vi "Find Scalar in Section.vi"(8 "error in":errorcluster, 10 "Scalar Data":T5, 11 "FPGA Addon refnum in":T2 format="%.0x") -> (0 "error out":errorcluster, 1 "Found ?":bool, 2 "Section Scalar Data":T1 {"Register Information"."Data Type" format="%.0x"; "Scalar Section ref" format="%.0x"}, 3 "FPGA Addon refnum out":T2=18446744073709551615 format="%.0x")   [LabVIEW 2018, in "Scripting API.lvlib"]
uses:
  Scripting API.lvlib
  <vilib>/NI Veristand/Custom Device API/Custom Device Item Ref.ctl
  TypeDefs/Input Scalar Data.ctl
  TypeDefs/Section Scalar Data.ctl
  Addon/Addon Shared/Types/Register Information.ctl
  Addon/Addon Shared/Types/FPGA Addon Data Type.ctl
  Addon/Addon Shared/Types/FG Action.ctl
  Addon/Addon Shared/SubVIs/Constants.vi
  <vilib>/NI/NI VeriStand Advanced SysDef API/_SubVIs/SysDef.Search.GUID.vi
  <vilib>/NI/NI VeriStand Advanced SysDef API/SysDef API/SysDef.Property.Get.vi
  <vilib>/NI/NI VeriStand Advanced SysDef API/_SubVIs/SysDef.Property.Get.Variant.vi
  <vilib>/NI/NI VeriStand Advanced SysDef API/SysDef API/SysDef.Property.Set.vi
  <vilib>/NI/NI VeriStand Advanced SysDef API/_SubVIs/SysDef.Property.Set.Variant.vi
  <vilib>/NI/NI VeriStand Advanced SysDef API/SysDef API/Advanced System Definition.lvlib
  Addon/Addon Shared/FPGA Addon Shared.lvlib
  <vilib>/NI Veristand/Custom Device API/Custom Device API.lvlib
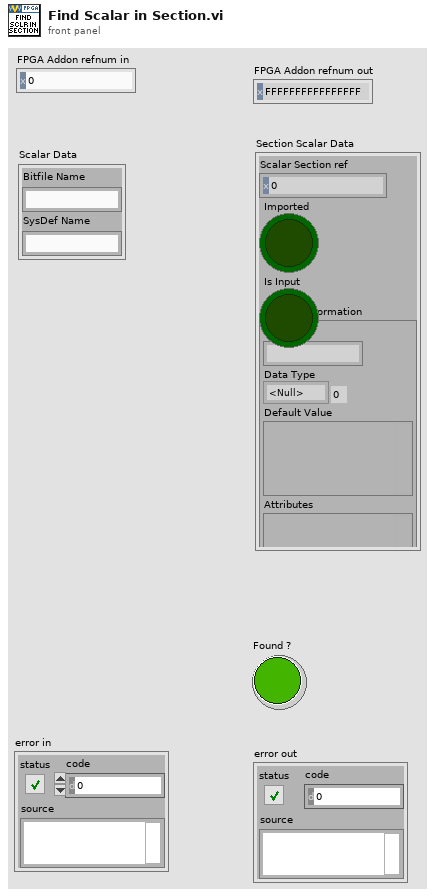
[diagram p1: front panel]
types:
  T1 = typedef "Scripting API.lvlib/Section Scalar Data.ctl" = cluster{"Scalar Section ref":T2, "Imported":bool, "Is Input":bool, "Register Information":T3}
  T2 = typedef "Custom Device API.lvlib/Custom Device Item Ref.ctl" = u64
  T3 = typedef "FPGA Addon Shared.lvlib/Register Information.ctl" = cluster{"Name":string, "Data Type":T4, "Default Value":variant, "Attributes":variant}
  T4 = typedef "FPGA Addon Shared.lvlib/FPGA Addon Data Type.ctl" = enum8{"<Null>", "I8", "I16", "I32", "I64", "U8", "U16", "U32", "U64", "SGL", "Boolean", "Analog PWM In Settings", "Analog PWM In", "Digital PWM In Settings", "Digital PWM In", "Digital PWM Out", "Sine Out", "FXP", "FXP+/-24.5", "FXP+/-16.5", "FXP+/-32.8", "FXP+/-64.32", "FXP+/-16.7", "FXP+/-20.5", "FXP+/-27.5", "FXP+/-32.16", "FXP+16.3", "FXP+18.3", "Digital Static In", "Digital Static Out", "Digital Static In Settings", "Digital WSS Out", "Quad Encoder Settings", "Quad Encoder In", "Group"}
  T5 = typedef "Scripting API.lvlib/Input Scalar Data.ctl" = cluster{"Bitfile Name":string, "SysDef Name":string}
  T6 = typedef "FPGA Addon Shared.lvlib/FG Action.ctl" = enum8{"GET", "SET"}
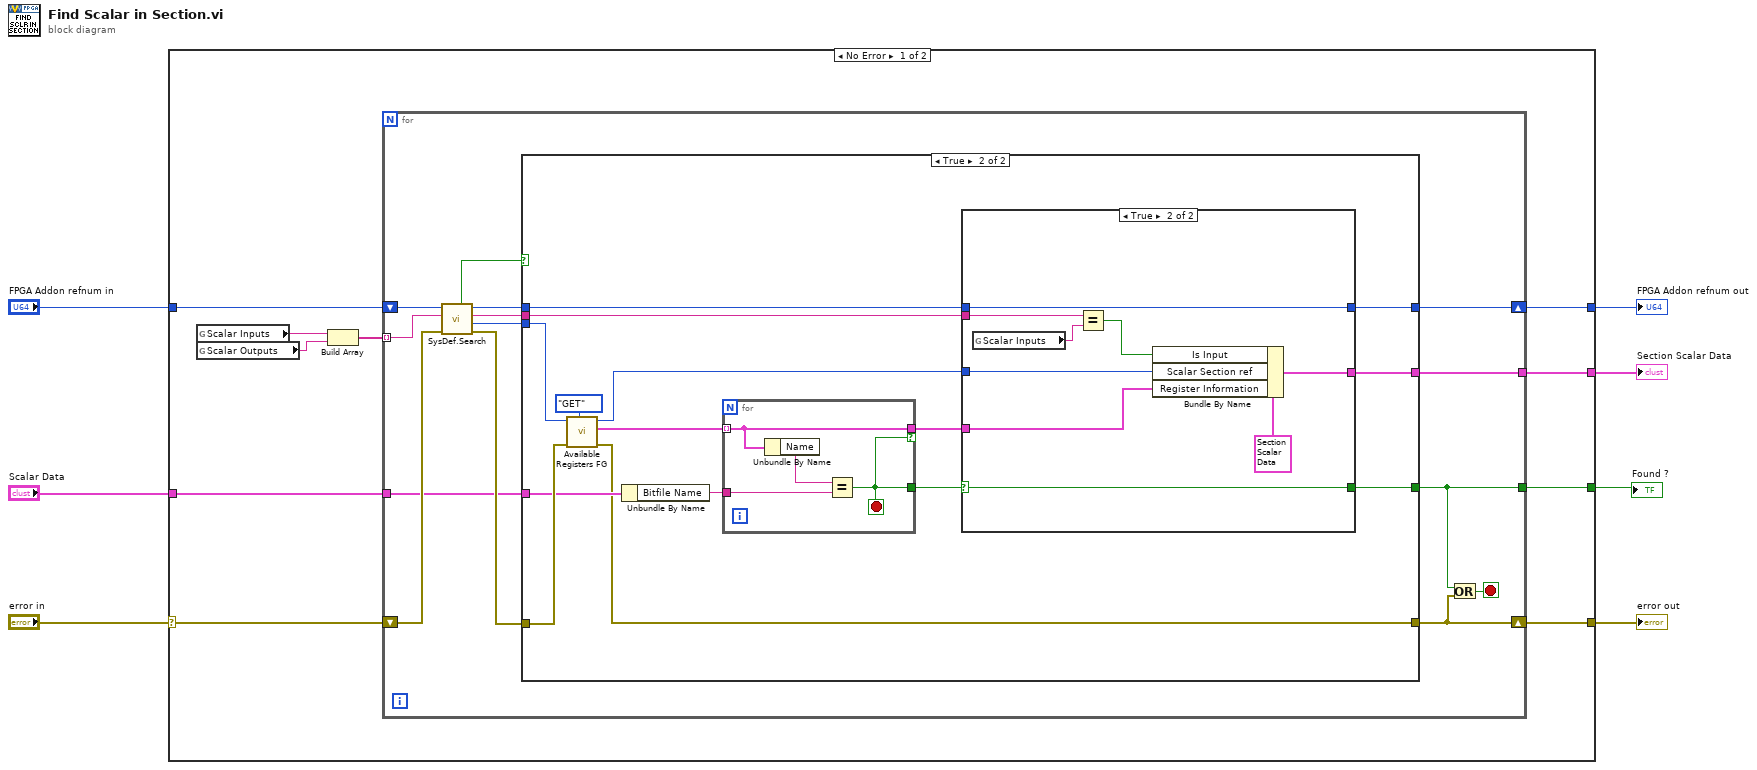
[diagram p0: block diagram]
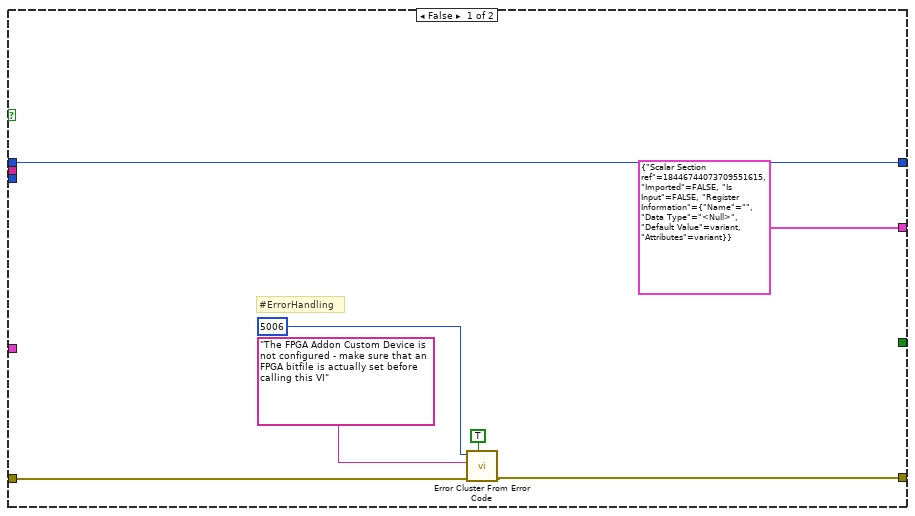
[diagram p2: hidden frame]
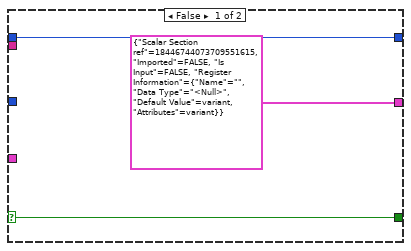
[diagram p3: hidden frame]
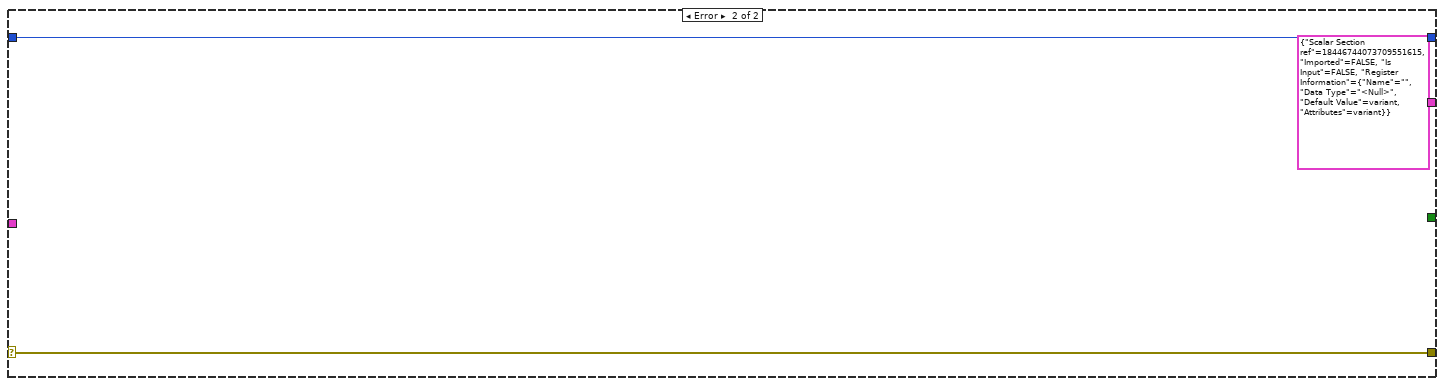
[diagram p4: hidden frame]
diagram:
  n1 = case shown="No Error" "error in" {
    selector: "error in" -> [w13 w71]
    tunnel: "FPGA Addon refnum in" -> [w14 w70]
    tunnel: [w12 w71] -> w5
    tunnel: [w11 w70] -> w4
    tunnel: "Scalar Data" -> [w10 _]
    tunnel: [w9 T1 {"Scalar Section ref"=18446744073709551615, "Imported"=FALSE, "Is Input"=FALSE, "Register Information"={"Name"="", "Data Type"=enum."<Null>", "Default Value"=variant, "Attributes"=variant}} ("Section Scalar Data")] -> w2
    tunnel: [w8 _] -> w1
    frame No Error {
      n2 = global read "Constants.vi" "Scalar Inputs"() -> (w16:string)
      n3 = global read "Constants.vi" "Scalar Outputs"() -> (w15:string)
      n4 = Build Array(w16, w15) -> (w17:string[])
      n5 = for {
        tunnel: w17 -> [w21] mode=indexing
        shift-right: [w26] -> w11
        shift-left: w14 -> [w30]
        shift-right: [w23] -> w12
        shift-left: w13 -> [w25]
        tunnel: w10 -> [w20]
        tunnel: [w19] -> w9
        tunnel: [w18] -> w8
        stop <- w22 stop-if-true
        n6 = call-poly <vilib>:"SysDef.Search.vi"("error in (no error)"=w25, "GUID"=w21, "nodeID"=w30) -> ("error out"=w24:errorcluster, "Value out"=w29:u64, "nodeID out"=w27:u64, "Found?"=w28:bool)  [unwired: 5 in]
        n7 = case shown="True" w28 {
          tunnel: w29 -> [_ w44]
          tunnel: w27 -> [w37 w42]
          tunnel: [w37 w41] -> w26
          tunnel: w24 -> [w32 w51]
          tunnel: [w31 w38] -> w23
          tunnel: w21 -> [_ w45]
          tunnel: w20 -> [_ w46]
          tunnel: [T1 {"Scalar Section ref"=18446744073709551615, "Imported"=FALSE, "Is Input"=FALSE, "Register Information"={"Name"="", "Data Type"=enum."<Null>", "Default Value"=variant, "Attributes"=variant}} ("Section Scalar Data") w40] -> w19
          tunnel: [_ w39] -> w18
          frame False {
            # "#ErrorHandling"
            n8 = call <vilib>:"Error Cluster From Error Code.vi"("show call chain? (False)"=TRUE, "error in (no error)"=w32, "error message (\"\")"="The FPGA Addon Custom Device is not configured - make sure that an FPGA bitfile is actually set before calling this VI" ("error message (\"\")"), "error code (0)"=5006) -> ("error out"=w31:errorcluster)  [unwired: 5 in]
          }
          frame True {
            n9 = call "Available Registers FG.vi"("Action"=FG_Action."GET", "error in (no error)"=w51, "Item Ref"=w44) -> ("error out"=w38:errorcluster, "Available Registers"=w50:T3[], "Item Ref out"=w43:T2)  [unwired: 6 in]
            n10 = Unbundle By Name(w46) -> ("Bitfile Name"=w49:string)
            n11 = for {
              tunnel: w50 -> [w66] mode=indexing
              tunnel: w49 -> [w67]
              tunnel: [w66] -> w47 if=w65
              tunnel: [w65] -> w48
              stop <- w65 stop-if-true
              n12 = Unbundle By Name(w66) -> ("Name"=w68:string)
              n13 = Equal?(x=w68, y=w67) -> (x = y?=w65:bool)
            }
            n14 = case shown="True" w48 {
              selector: w48 -> [w55 w57]
              tunnel: w47 -> [_ w59]
              tunnel: w45 -> [_ w62]
              tunnel: w43 -> [_ w63]
              tunnel: w42 -> [w54 w58]
              tunnel: [w54 w58] -> w41
              tunnel: [w55 w57] -> w39
              tunnel: [T1 {"Scalar Section ref"=18446744073709551615, "Imported"=FALSE, "Is Input"=FALSE, "Register Information"={"Name"="", "Data Type"=enum."<Null>", "Default Value"=variant, "Attributes"=variant}} ("Section Scalar Data") w56] -> w40
              frame False {
              }
              frame True {
                n15 = global read "Constants.vi" "Scalar Inputs"() -> (w61:string)
                n16 = Equal?(x=w62, y=w61) -> (x = y?=w60:bool)
                n17 = Bundle By Name(cluster=T1 {"Scalar Section ref"=0, "Imported"=FALSE, "Is Input"=FALSE, "Register Information"={"Name"="", "Data Type"=enum."<Null>", "Default Value"=variant, "Attributes"=variant}} ("Section Scalar Data"), "Is Input"=w60, "Scalar Section ref"=w63, "Register Information"=w59) -> (w56:T1)
              }
            }
          }
        }
        n18 = Or(x=w18, y=w23) -> (x .or. y?=w22:bool)
      }
    }
    frame Error {
    }
  }
  "error out" <- w5
  "FPGA Addon refnum out" <- w4
  "Found ?" <- w1
  "Section Scalar Data" <- w2
